vi "posição da borboleta(SubVI).vi"(11 "data in":string) -> (3 "Numeric":dbl)   [LabVIEW 2015]
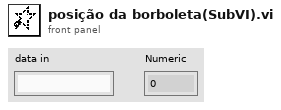
[diagram p1: front panel]
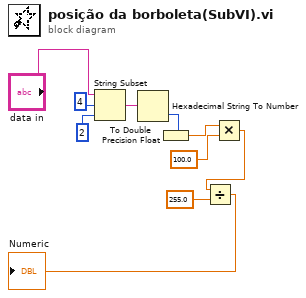
[diagram p0: block diagram]
diagram:
  n1 = String Subset(string="data in", offset (0)=4, length (rest)=2 ("length (rest)")) -> (substring=w5:string)
  n2 = Hexadecimal String To Number(string=w5) -> (number=w6:u32)  [unwired: 2 in, 1 out]
  n3 = To Double Precision Float(number=w6) -> (double precision float=w8:dbl)
  n4 = Multiply(x=w8, y=100.0) -> (x*y=w1:dbl)
  n5 = Divide(x=w1, y=255.0) -> (x/y=→"Numeric":dbl)
